vi "ShouldLog.vi"(8 "error in (no error)":errorcluster, 10 "LogRecord":refnum<class "LogRecord.lvclass">, 11 "FileHandler in":refnum<class "RotateFileHandler.lvclass">) -> (0 "error out":errorcluster, 1 "Log?":bool, 2 "LogRecord out":refnum<class "LogRecord.lvclass">, 3 "FileHandler out":refnum<class "RotateFileHandler.lvclass">)   [LabVIEW 2024, in "RotateFileHandler.lvclass"]
uses:
  RotateFileHandler.lvclass
  <vilib>/Hampel Software Engineering/HSE Logger/LogRecord/LogRecord.lvclass
  <vilib>/Hampel Software Engineering/HSE Logger/LogRecord/LogRecord.lvclass/LogRecord.ctl
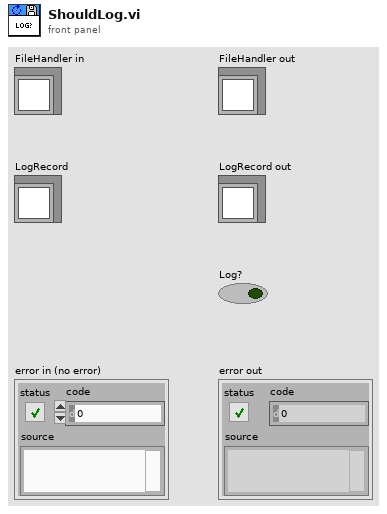
[diagram p1: front panel]
types:
  T1 = typedef "hse-logger.lvlib/LogLevel.ctl" = enum16{"DEBUG", "INFO", "WARNING", "ERROR", "CRITICAL"}
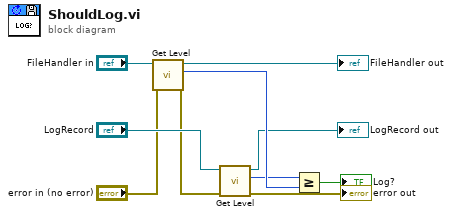
[diagram p0: block diagram]
diagram:
  n1 = call-dynamic <vilib>:"Get Level.vi"("error in"="error in (no error)", "Handler in"="FileHandler in") -> ("error out"=w2:errorcluster, "Level"=w8:T1, "Handler out"=→"FileHandler out":refnum<class "RotateFileHandler.lvclass">)  [unwired: 7 in]
  n2 = call <vilib>:"Get Level.vi"("error in"=w2, "LogRecord in"="LogRecord") -> ("error out"=→"error out":errorcluster, "Level"=w7:T1, "LogRecord out"=→"LogRecord out":refnum<class "LogRecord.lvclass">)  [unwired: 7 in]
  n3 = Greater Or Equal?(x=w7, y=w8) -> (x >= y?=→"Log?":bool)
